vi "HWIO Global.vi"() -> ()   [LabVIEW 2011]
panel:
  in  "API Token":string
  in  "API Port":u16=80
  in  "API Server":string="localhost"
  in  "CONNECTION":refnum<k5>
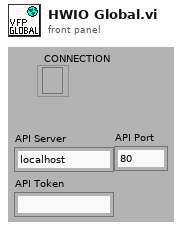
[diagram p1: front panel]
diagram:
